vi "ImageClickDetect.vi"(5 "Change":refnum<vi>, 7 "Stop":refnum<vi>, 9 "Mouse Point":refnum<vi>, 11 "image Ref String":string) -> ()   [LabVIEW 2014]
panel:
  out "ImXY_Point":i32[](array[numeric])
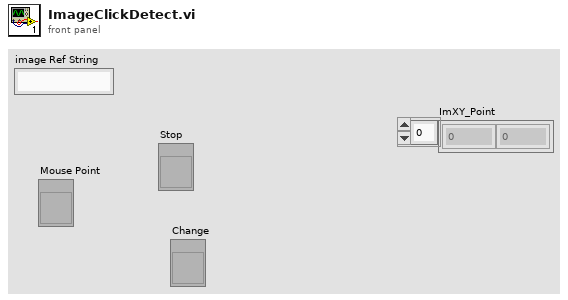
[diagram p1: front panel]
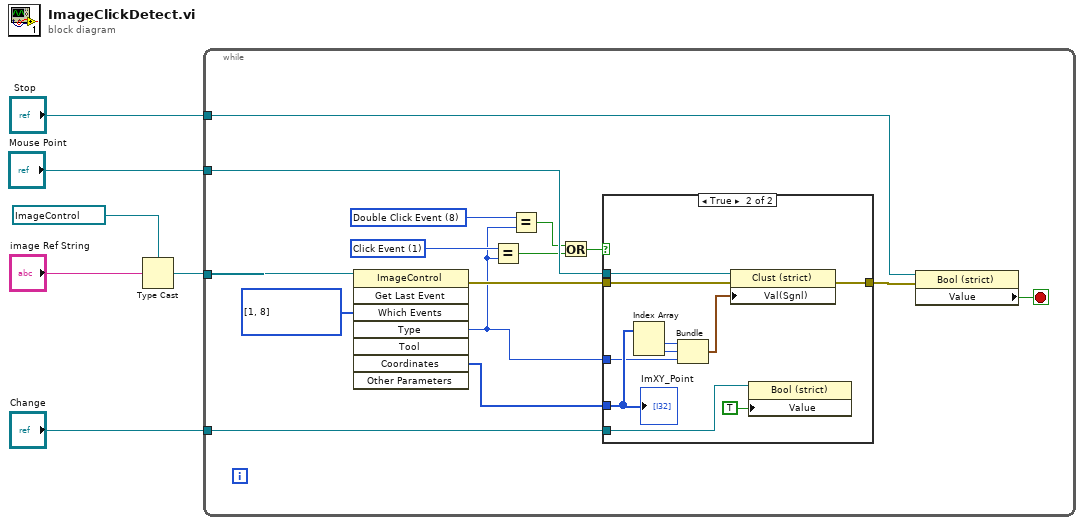
[diagram p0: block diagram]
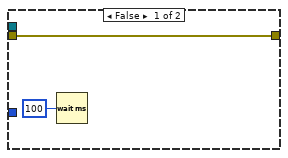
[diagram p2: hidden frame]
diagram:
  n1 = Type Cast(type=refnum<vi> refnum ("Image"), x="image Ref String") -> (*(type *) &x=w4:refnum<vi>)
  n2 = while {
    tunnel: w4 -> [w21]
    tunnel: "Stop" -> [w17]
    tunnel: "Mouse Point" -> [w15]
    tunnel: "Change" -> [w12]
    stop <- w16 stop-if-true
    w11 = 8 items=["No Event"=0, "Click Event"=1, "Draw Event"=2, "Size Event"=4, "Scroll Event"=5, "Double Click Event"=8]
    w19 = 1 items=["No Event"=0, "Click Event"=1, "Draw Event"=2, "Size Event"=4, "Scroll Event"=5, "Double Click Event"=8]
    w20 = i32[] [1, 8] items=["No Event"=0, "Click Event"=1, "Draw Event"=2, "Size Event"=4, "Scroll Event"=5, "Double Click Event"=8] ("Which Events")
    n3 = invoke class="ImageControl" method="Get Last Event"(reference=w21, "Which Events"=w20) -> (error out=w14:errorcluster, "Type"=w7:i32, "Coordinates"=w18:i32[])  [unwired: 6 in, 5 out]
    n4 = Equal?(x=w19, y=w7) -> (x = y?=w8:bool)
    n5 = Equal?(x=w11, y=w7) -> (x = y?=w9:bool)
    n6 = Or(x=w9, y=w8) -> (x .or. y?=w10:bool)
    n7 = case shown="True" w10 {
      tunnel: w18 -> [_ w30]
      tunnel: w15 -> [_ w33]
      tunnel: w14 -> [w22 w32]
      tunnel: [w22 w31] -> w13
      tunnel: w12 -> [_ w26]
      tunnel: w7 -> [_ w25]
      frame False {
        n8 = Wait (ms)(milliseconds to wait=u32 100) -> ()  [unwired: 1 out]
      }
      frame True {
        n9 = Index Array(array=w30) -> (element #1=w29:i32, element #2=w28:i32)  [unwired: 2 in]
        n10 = Bundle(w29, w28, "Type"=w25) -> (w24:cluster{i32, i32, "Type":i32})  [unwired: 1 in]
        n11 = property class="Clust (strict)"(reference=w33, error in=w32, "Val(Sgnl)"=w24) -> (error out=w31:errorcluster)  [unwired: 1 out]
        n12 = property class="Bool (strict)"(reference=w26, "Value"=TRUE ("Boolean")) -> ()  [unwired: 1 in, 2 out]
        "ImXY_Point" <- w30
      }
    }
    n13 = property class="Bool (strict)"(reference=w17, error in=w13) -> ("Value"=w16:bool)  [unwired: 2 out]
  }
